vi "Run.vi"(8 "error in (no error)":errorcluster, 11 "AM-AM in":refnum<class "AM-AM.lvclass">) -> (0 "error out":errorcluster, 1 "Parameters":cluster{"Name":string, "Value":string}[](array[cluster]), 2 "Cancled":bool, 3 "AM-AM out":refnum<class "AM-AM.lvclass">)   [LabVIEW 2020, in "AM-AM.lvclass"]
doc: "This is the main test vi. It is here that the test is implemented."
uses:
  AM-AM.lvclass
  C:/Sandbox/RF Bench/Source Code/WiSpry Test Framework/Measurements/Measurement.lvclass
  Controls/Run states.ctl
  Controls/Loop order.ctl
  AM-AM.lvclass/AM-AM.ctl
  Instruments/Spectrum Analyzer/Spectrum Analyzer.lvclass/Spectrum Analyzer.ctl
  Measurement.lvclass/Measurement.ctl
  Devices/Controls/Change setting mode enum.ctl
  Support VI/Update parameters (single).vi
  Devices/Device.lvclass
  Instruments/Spectrum Analyzer/Spectrum Analyzer.lvclass
  Instruments/Signal Generator/Signal Generator.lvclass
  Instruments/Power Meter/Power Meter.lvclass
  Measurement.lvclass
  Devices/PIC-device/PIC-Device.lvclass
  XML Handler/XML Handler.lvclass
panel:
  out "Device Parameters":string
  out "Current Power [dBm]":dbl
  out "Current Frequency [Hz]":dbl format="%#_6p"
  out "Progress":u8(slide) scale=0.0..100.0
  in  "Cancel Button":bool
  out "XY Graph":cluster{dbl[], dbl[]}[](graph)
  out "Estimated finish time":timestamp format="%<%X>T"
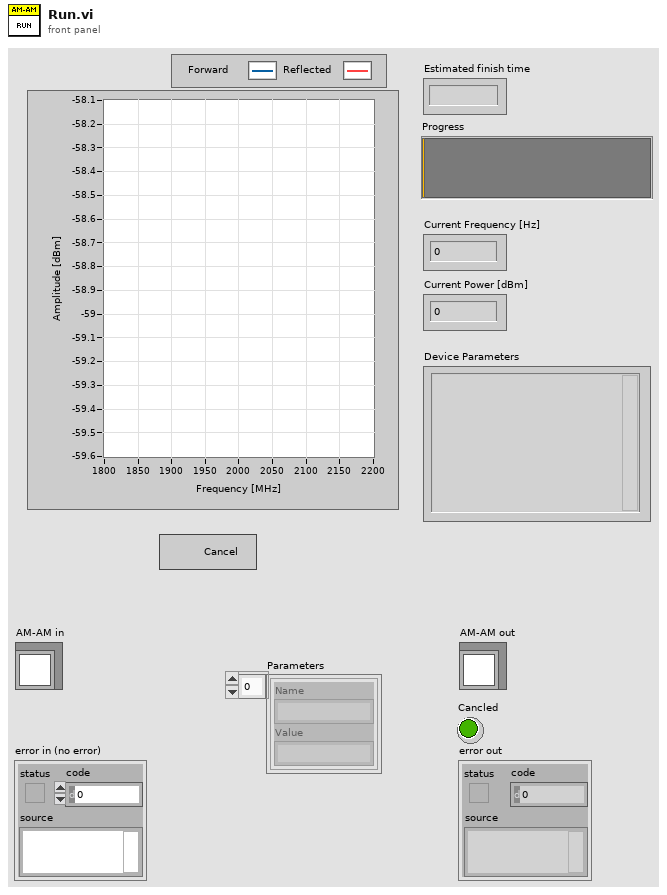
[diagram p1: front panel]
types:
  T1 = typedef "AM-AM.lvclass/Loop order.ctl" = enum16{"Device -> Power -> Frequency", "Device -> Frequency -> Power"}
  T2 = typedef "AM-AM.lvclass/Run states.ctl" = enum16{"Init", "Set Device", "Set Power", "Set Frequency", "Measure", "Done"}
  T3 = typedef "PIC-Device.lvclass/Change setting mode enum.ctl" = enum16{"Init", "Next", "Reset"}
  T4 = typedef "AM-AM.lvclass/Config info.ctl" = cluster{"RBW":dbl, "VBW ":dbl, "Number of Averages":dbl, "Average On":bool, "Power":cluster{"Cluster ":cluster{"From":dbl, "To":dbl, "Step":dbl}, "Array":dbl[], "Use Array":bool}, "Frequency":cluster{"Cluster ":cluster{"From":dbl, "To":dbl, "Step":dbl}, "Array":dbl[], "Use Array":bool}, "Loop order":T1, "Power Window":dbl}
  T5 = typedef "XML Handler.lvclass/Result Cluster.ctl" = cluster{"Name":string, "Value":string}
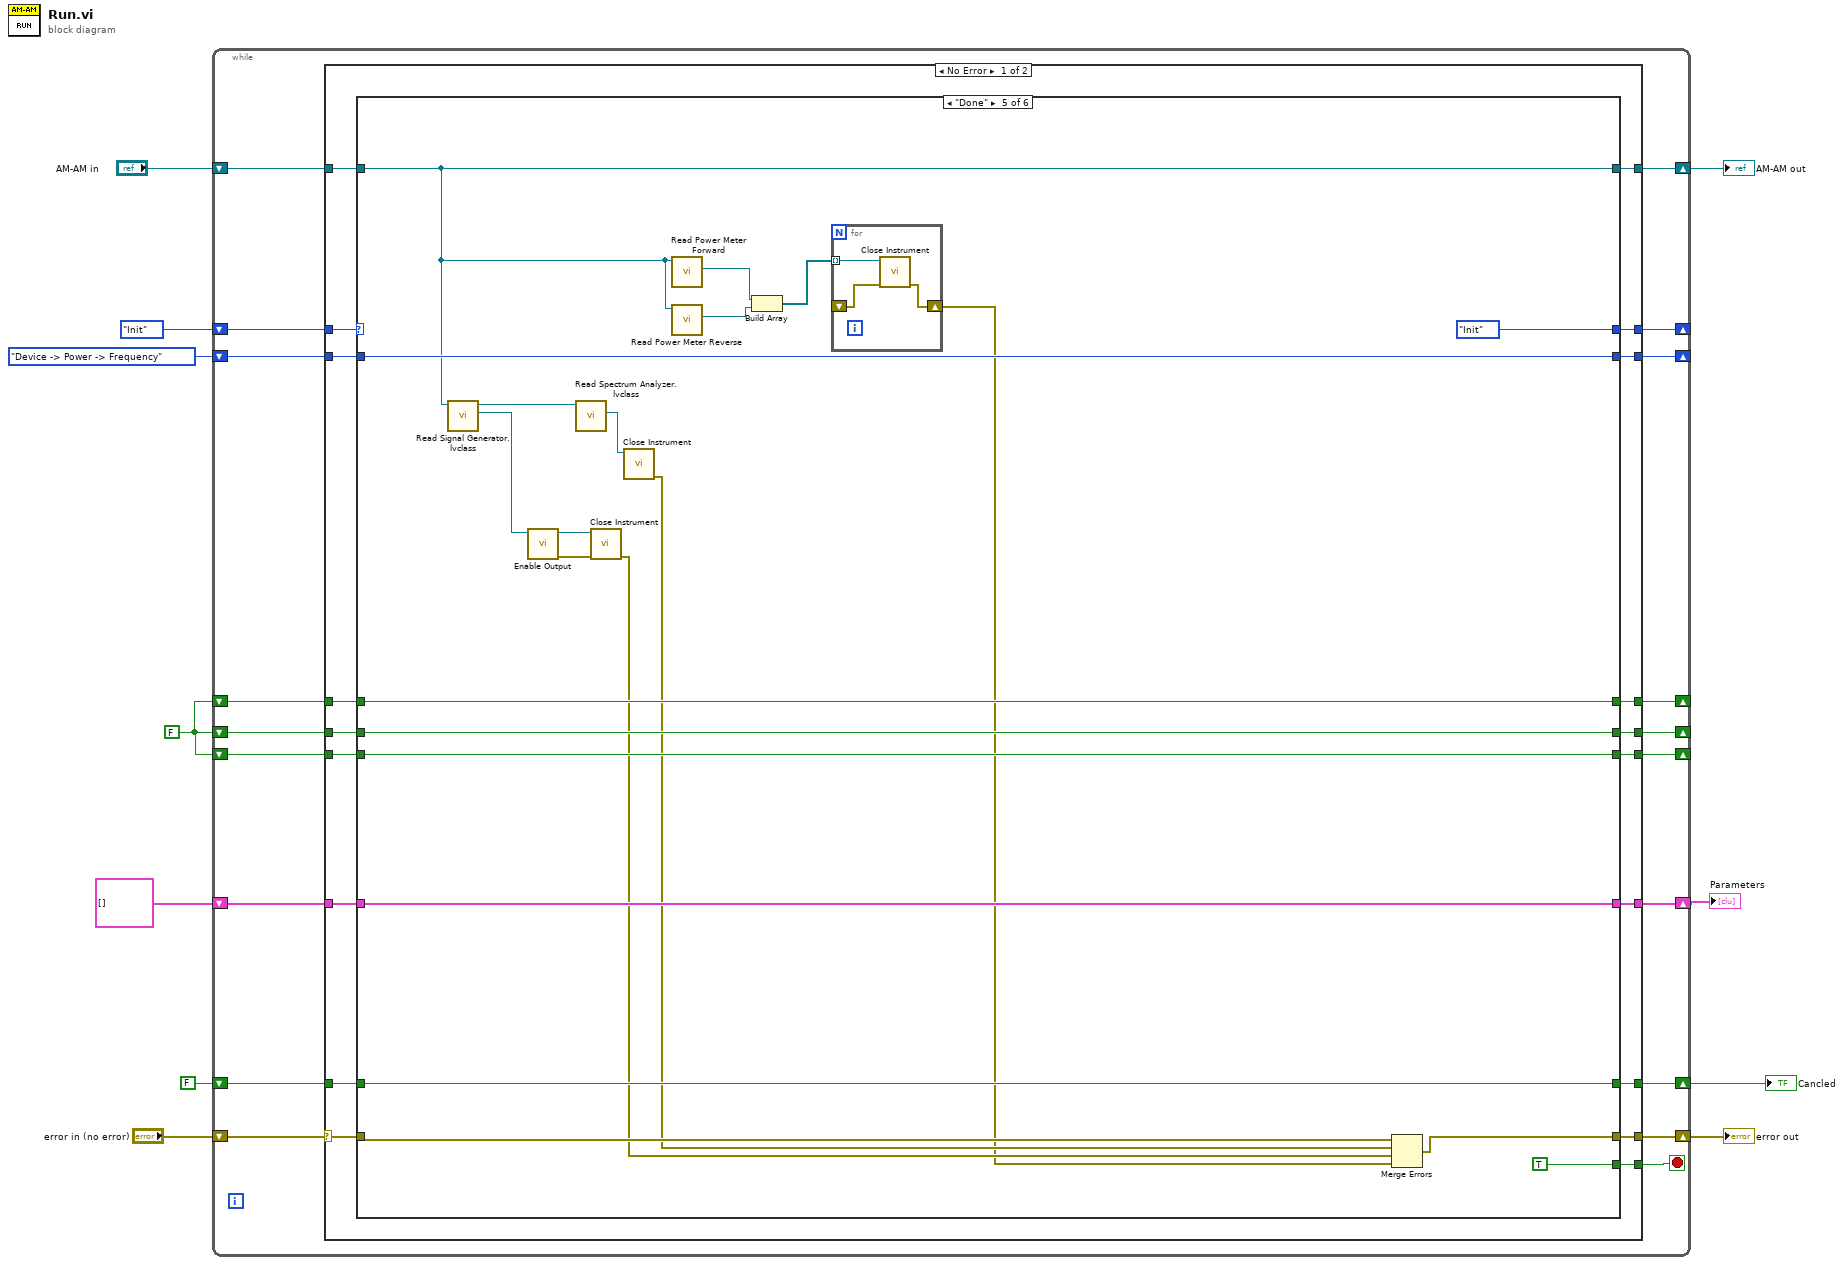
[diagram p0: block diagram]
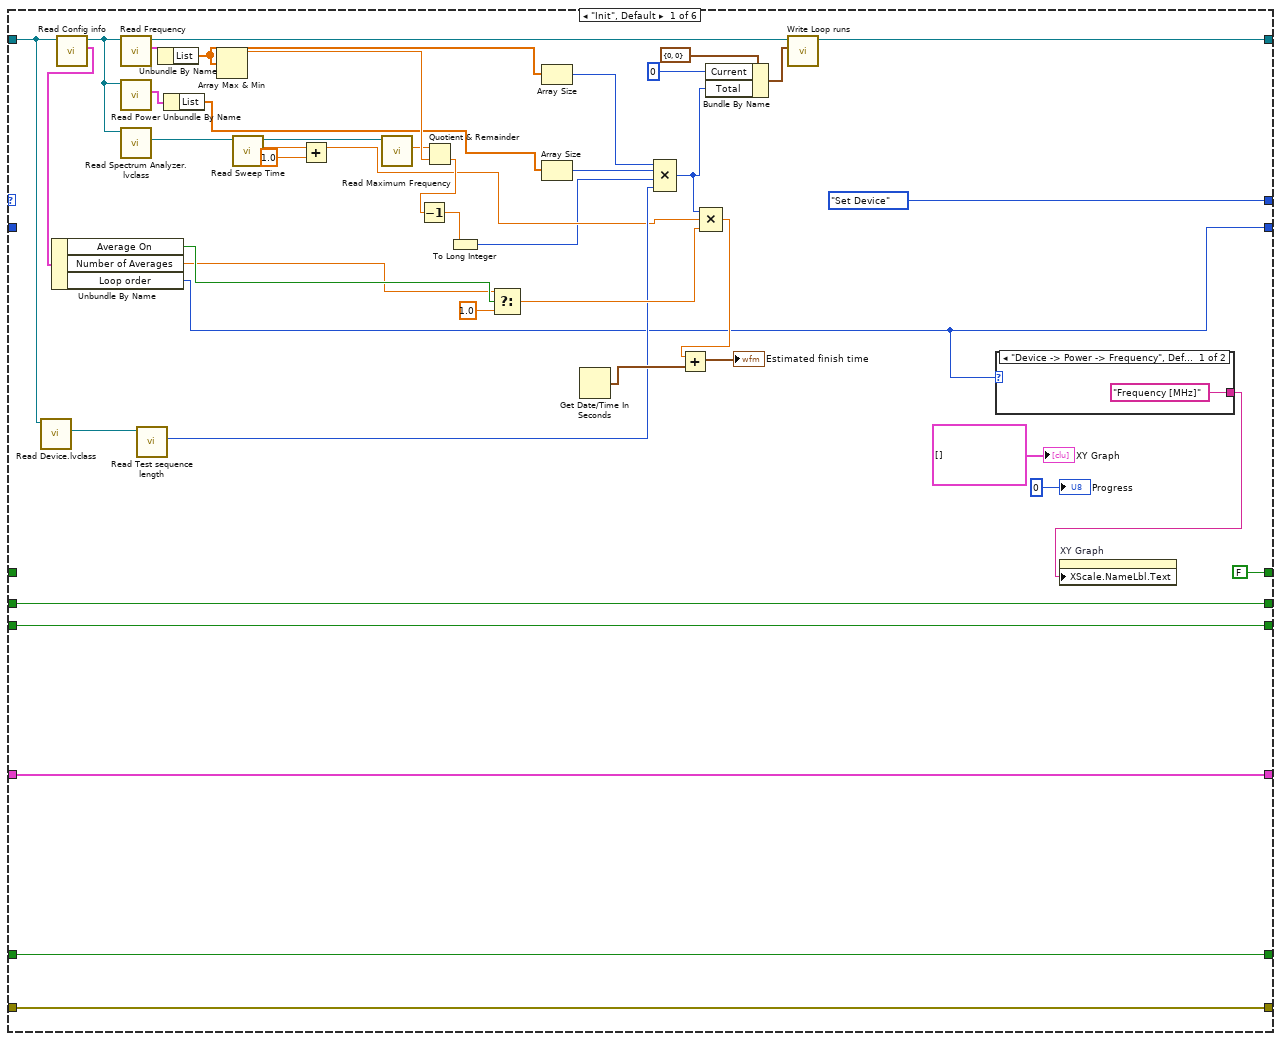
[diagram p2: hidden frame]
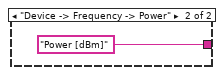
[diagram p3: hidden frame]
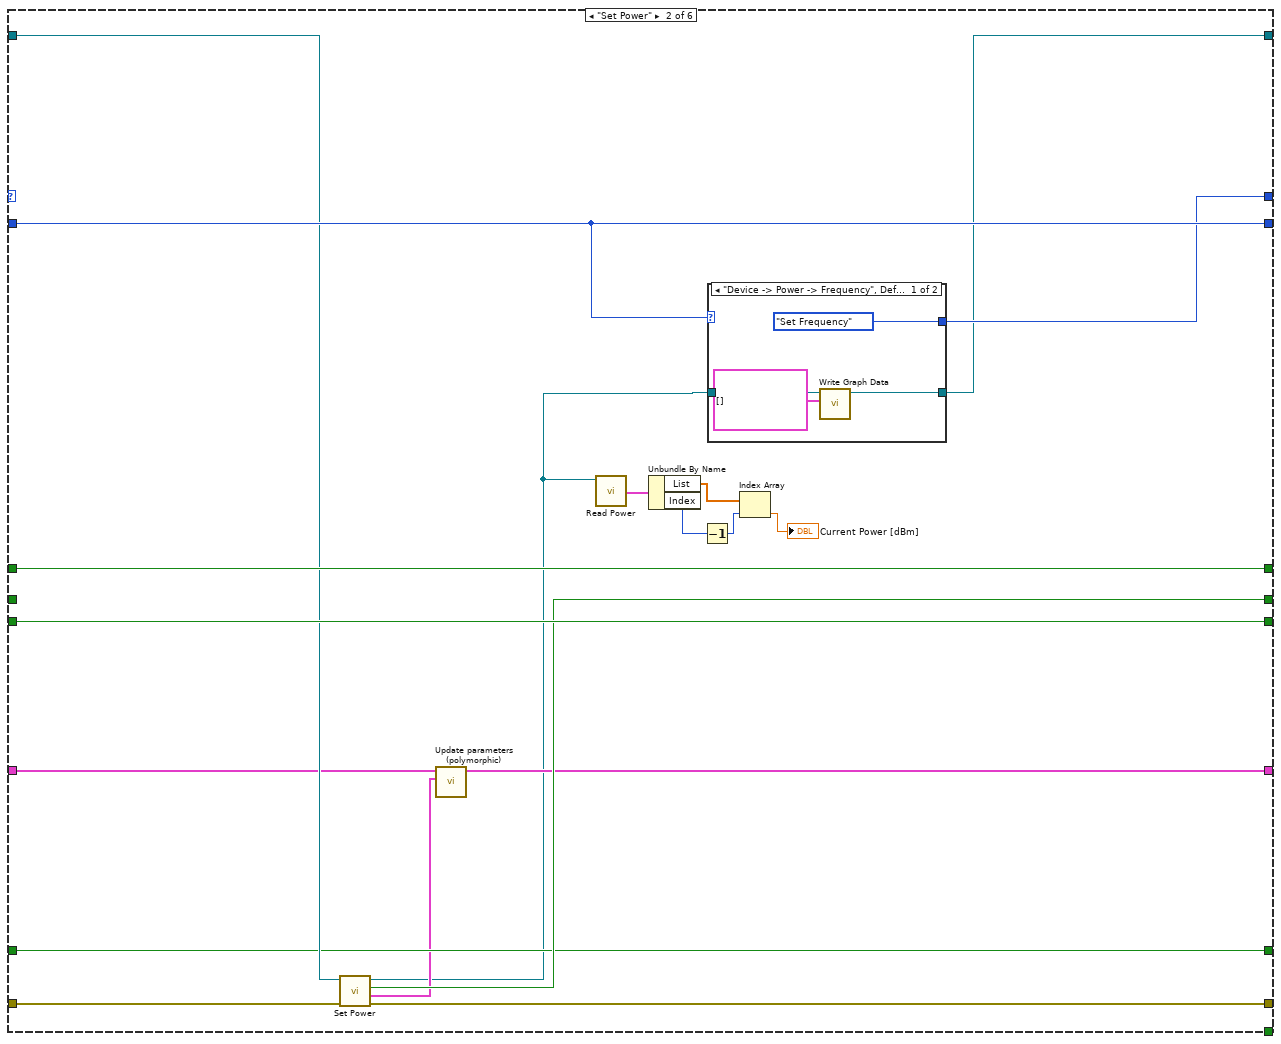
[diagram p4: hidden frame]
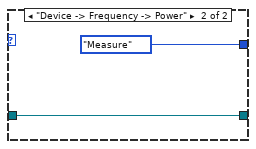
[diagram p5: hidden frame]
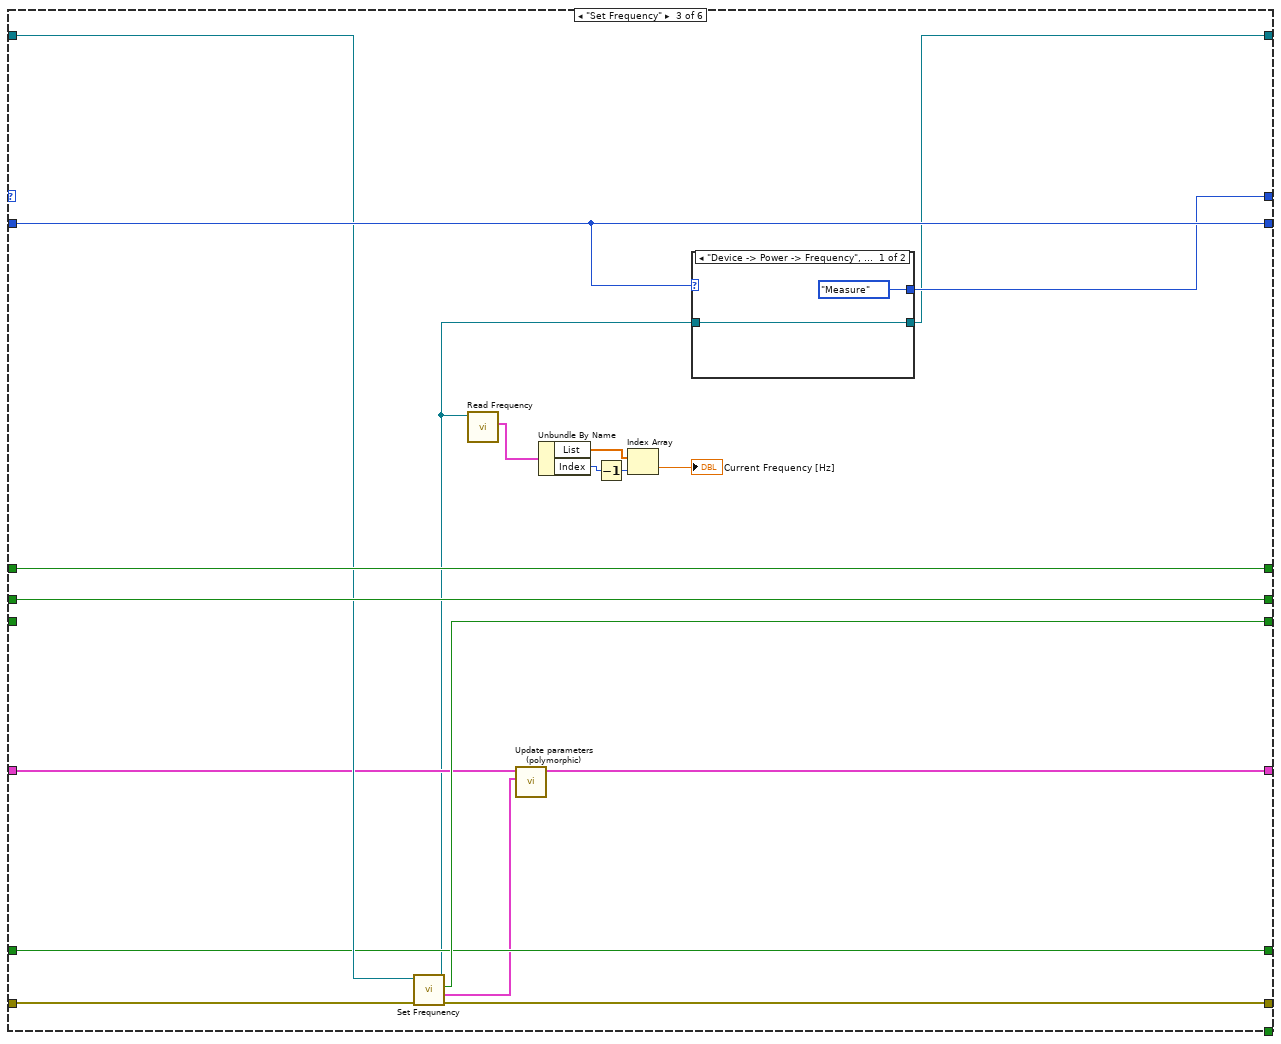
[diagram p6: hidden frame]
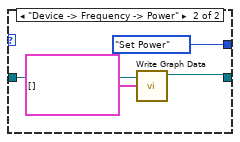
[diagram p7: hidden frame]
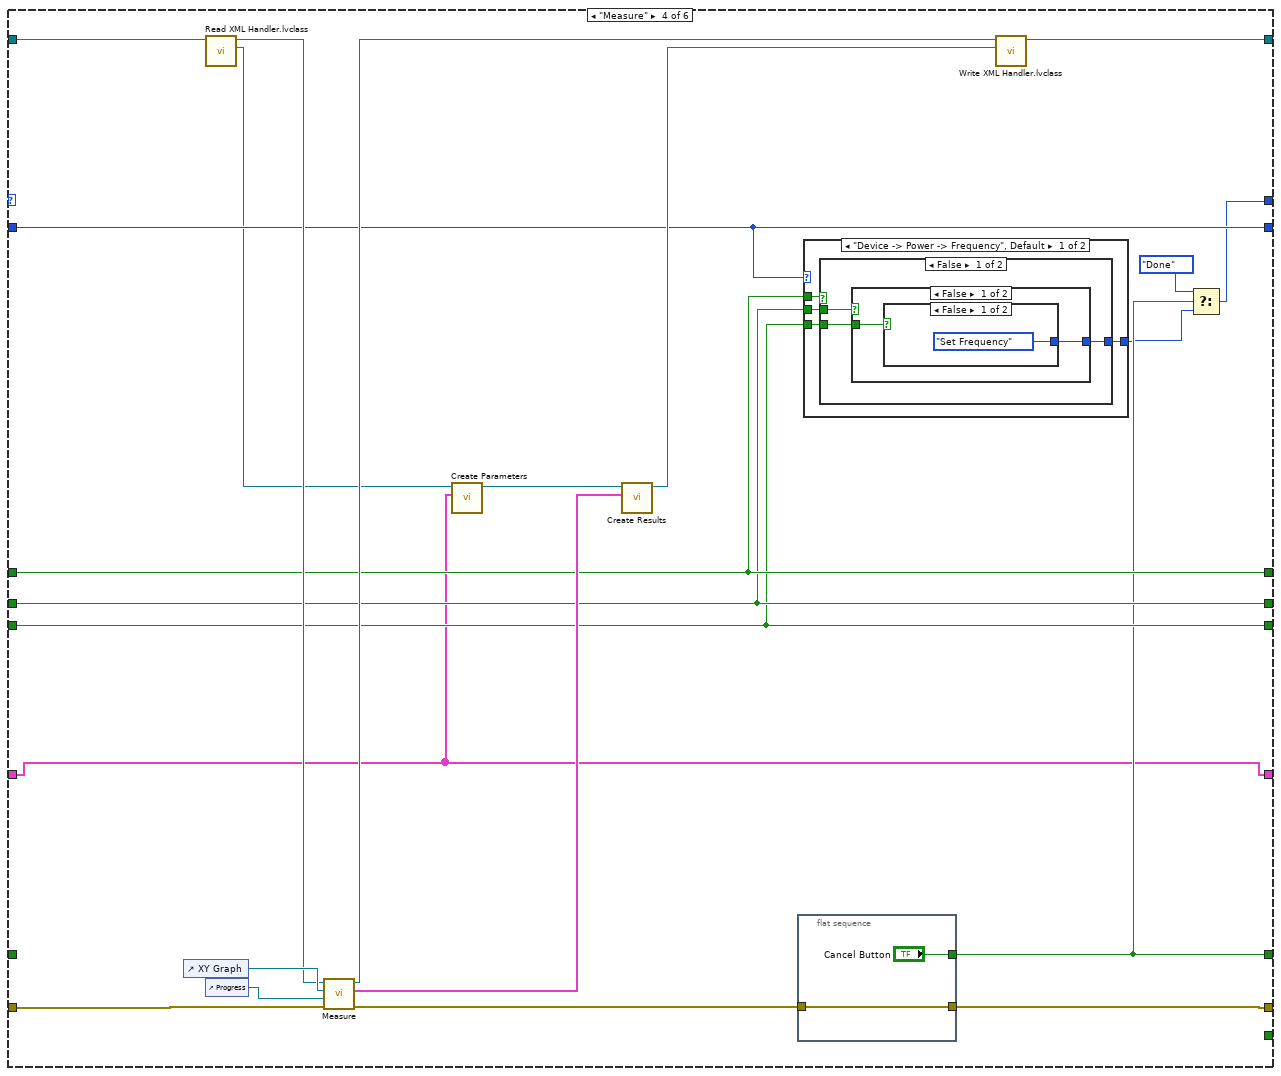
[diagram p8: hidden frame]
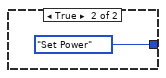
[diagram p9: hidden frame]
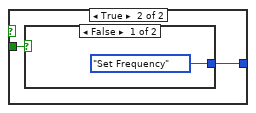
[diagram p10: hidden frame]
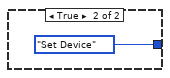
[diagram p11: hidden frame]
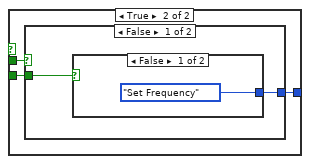
[diagram p12: hidden frame]
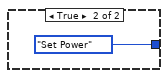
[diagram p13: hidden frame]
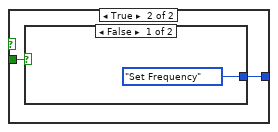
[diagram p14: hidden frame]
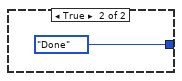
[diagram p15: hidden frame]
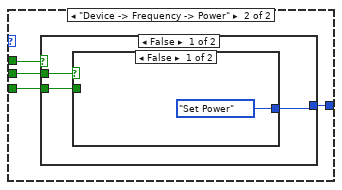
[diagram p16: hidden frame]
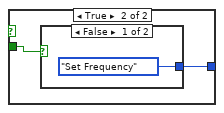
[diagram p17: hidden frame]
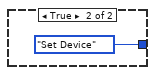
[diagram p18: hidden frame]
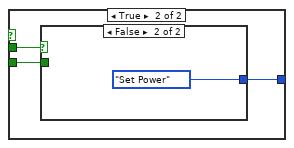
[diagram p19: hidden frame]
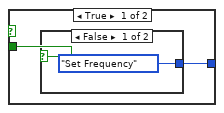
[diagram p20: hidden frame]
diagram:
  w6 = FALSE
  n1 = while {
    shift-right: [w25] -> w8
    shift-left: "error in (no error)" -> [w30]
    shift-right: [w27] -> w9
    shift-left: "AM-AM in" -> [w29]
    shift-right: [w22] -> _
    shift-left: Run_states."Init" ("Run states") -> [w28]
    shift-right: [w24] -> _
    shift-left: w6 -> [w23]
    shift-right: [w21] -> _
    shift-left: Loop_order."Device -> Power -> Frequency" ("Loop order") -> [w20]
    shift-right: [w17] -> _
    shift-left: w6 -> [w19]
    shift-right: [w16] -> _
    shift-left: w6 -> [w18]
    shift-right: [w15] -> w4
    shift-left: FALSE ("Cancel Button") -> [w14]
    shift-right: [w12] -> w1
    shift-left: cluster{"Name":string, "Value":string}[] [] ("Parameters") -> [w13]
    stop <- w26 stop-if-true
    n2 = case shown="No Error" w30 {
      selector: w30 -> [w46 w280]
      tunnel: w29 -> [w49 w281]
      tunnel: w28 -> [w48 _]
      tunnel: [w47 w281] -> w27
      tunnel: [w45 TRUE] -> w26
      tunnel: [w44 w280] -> w25
      tunnel: [w43 _] -> w24
      tunnel: w23 -> [w42 _]
      tunnel: [w41 _] -> w22
      tunnel: [w40 _] -> w21
      tunnel: w20 -> [w39 _]
      tunnel: w19 -> [w38 _]
      tunnel: w18 -> [w37 _]
      tunnel: [w36 _] -> w17
      tunnel: [w35 _] -> w16
      tunnel: [w34 _] -> w15
      tunnel: w14 -> [w33 _]
      tunnel: w13 -> [w32 w279]
      tunnel: [w31 w279] -> w12
      frame No Error {
        n3 = case shown="\"Done\"" w48 {
          tunnel: w49 -> [w79 w110 w135 w166 w220 w266]
          tunnel: [w51 w107 w132 w161 w220 w254] -> w47
          tunnel: w46 -> [w55 w111 w136 w168 w225 w263]
          tunnel: [_ _ _ _ TRUE _] -> w45
          tunnel: [w55 w106 w131 w159 w222 w251] -> w44
          tunnel: [FALSE ("Last setting") w115 w140 w157 w237 w261] -> w43
          tunnel: w42 -> [_ w115 w140 w157 w237 _]
          tunnel: [Run_states."Set Device" ("Run states") w113 w138 w151 Run_states."Init" ("Run states") w257] -> w41
          tunnel: [w57 w114 w139 w158 w238 w258] -> w40
          tunnel: w39 -> [_ w114 w139 w158 w238 w258]
          tunnel: w38 -> [w72 _ w137 w156 w236 w260]
          tunnel: w37 -> [w71 w112 _ w155 w235 w259]
          tunnel: [w72 w109 w137 w156 w236 w260] -> w36
          tunnel: [w71 w112 w134 w155 w235 w259] -> w35
          tunnel: [w66 w108 w133 w154 w232 w256] -> w34
          tunnel: w33 -> [w66 w108 w133 _ w232 w256]
          tunnel: w32 -> [w60 w105 w130 w147 w230 w250]
          tunnel: [w60 w104 w129 w147 w230 w246] -> w31
          frame "Init", Default {
            n4 = call "Read Device.lvclass.vi"("Measurements in"=w79) -> ("Device.lvclass"=w74:refnum<class "Device.lvclass">)  [unwired: 9 in, 1 out]
            n5 = call "Read Config info.vi"("AM-AM in"=w79) -> ("Config info"=w93:T4, "AM-AM out"=w94:refnum<class "AM-AM.lvclass">)  [unwired: 9 in]
            n6 = Unbundle By Name(w93) -> ("Average On"=w84:bool, "Number of Averages"=w83:dbl, "Loop order"=w57:T1)
            n7 = call "Read Frequency.vi"("AM-AM in"=w94) -> ("Frequency"=w70:cluster{"List":dbl[], "Index":i32, "Last":bool}, "AM-AM out"=w65:refnum<class "AM-AM.lvclass">)  [unwired: 9 in]
            n8 = call "Read Power.vi"("AM-AM in"=w94) -> ("Power"=w68:cluster{"List":dbl[], "Index":i32, "Last":bool})  [unwired: 9 in, 1 out]
            n9 = call "Read Spectrum Analyzer.lvclass.vi"("AM-AM in"=w94) -> ("Spectrum Analyzer.lvclass"=w92:refnum<class "Spectrum Analyzer.lvclass">)  [unwired: 9 in, 1 out]
            n10 = call-dynamic "Read Test sequence length.vi"("Device in"=w74) -> ("Test sequence length"=w75:i32)  [unwired: 8 in, 2 out]
            n11 = Unbundle By Name(w70) -> ("List"=w69:dbl[])
            n12 = Unbundle By Name(w68) -> ("List"=w67:dbl[])
            n13 = Array Max & Min(array=w69) -> (max value=w90:dbl)  [unwired: 3 out]
            n14 = call "Read Sweep Time.vi"("Spectrum Analyzer in"=w92) -> ("Sweep Time"=w87:dbl, "Spectrum Analyzer out"=w91:refnum<class "Spectrum Analyzer.lvclass">)  [unwired: 9 in]
            n15 = Add(x=w87, y=1.0) -> (x+y=w53:dbl)
            n16 = call "Read Maximum Frequency.vi"("Spectrum Analyzer in"=w91) -> ("Maximum Frequency"=w89:dbl)  [unwired: 9 in, 1 out]
            n17 = Quotient & Remainder(x=w89, y=w90) -> (floor(x/y)=w88:dbl)  [unwired: 1 out]
            n18 = Decrement(x=w88) -> (x-1=w80:dbl)
            n19 = To Long Integer(number=w80) -> (32bit integer=w50:i32)
            n20 = Select(t=w83, s=w84, f=1.0) -> (s? t:f=w81:dbl)
            n21 = Array Size(array=w69) -> (size(s)=w77:i32)
            n22 = Array Size(array=w67) -> (size(s)=w76:i32)
            n23 = Get Date/Time In Seconds() -> (seconds since 1Jan1904=w86:timestamp)
            n24 = Compound Arithmetic op=MULTIPLY(w77, w76, w50, w75) -> (w61:i32)
            n25 = Compound Arithmetic op=MULTIPLY(w61, w53, w81) -> (w78:dbl)
            n26 = Add(x=w78, y=w86) -> (x+y=→"Estimated finish time":timestamp)
            n27 = Bundle By Name(cluster=cluster{"Current":u32, "Total":u32} {"Current"=0, "Total"=0} ("Loop runs"), "Current"=u32 0, "Total"=w61) -> (w62:cluster{"Current":u32, "Total":u32})
            n28 = call "Write Loop runs.vi"("Loop runs"=w62, "Measurements in"=w65) -> ("Measurements out"=w51:refnum<class "AM-AM.lvclass">)  [unwired: 9 in]
            n29 = case shown="\"Device -> Power -> Frequency\", Default" w57 {
              tunnel: ["Frequency [MHz]" "Power [dBm]"] -> w56
              frame "Device -> Power -> Frequency", Default {
              }
              frame "Device -> Frequency -> Power" {
              }
            }
            n30 = property on="XY Graph" class="XYGraph (strict)"("XScale.NameLbl.Text"=w56) -> ()  [unwired: 2 in, 2 out]
            "XY Graph" <- cluster{dbl[], dbl[]}[] [] ("XY Graph")
            "Progress" <- u8 0 ("Progress")
          }
          frame "Set Power" {
            n31 = call "Set Power.vi"("error in (no error)"=w111, "AM-AM in"=w110) -> ("error out"=w106:errorcluster, "Parameter"=w103:cluster{"Name":string, "Value":string}, "Last Power?"=w109:bool, "AM-AM out"=w102:refnum<class "AM-AM.lvclass">)  [unwired: 6 in]
            n32 = call-poly "Update parameters (polymorphic).vi"("New Parameter"=w103, "Parameters"=w105) -> ("Parameters Out"=w104:cluster{"Name":string, "Value":string}[])  [unwired: 9 in]
            n33 = call "Read Power.vi"("AM-AM in"=w102) -> ("Power"=w101:cluster{"List":dbl[], "Index":i32, "Last":bool})  [unwired: 9 in, 1 out]
            n34 = Unbundle By Name(w101) -> ("List"=w99:dbl[], "Index"=w97:i32)
            n35 = Decrement(x=w97) -> (x-1=w98:i32)
            n36 = case shown="\"Device -> Power -> Frequency\", Default" w114 {
              tunnel: [Run_states."Set Frequency" ("Run states") Run_states."Measure" ("Run states")] -> w113
              tunnel: w102 -> [w118 w120]
              tunnel: [w117 w120] -> w107
              frame "Device -> Power -> Frequency", Default {
                n37 = call "Write Graph Data.vi"("Graph Data"=cluster{"Array":dbl[], "Array":dbl[]}[] [], "AM-AM in"=w118) -> ("AM-AM out"=w117:refnum<class "AM-AM.lvclass">)  [unwired: 9 in]
              }
              frame "Device -> Frequency -> Power" {
              }
            }
            n38 = Index Array(array=w99, index=w98) -> (element=→"Current Power [dBm]":dbl)
          }
          frame "Set Frequency" {
            n39 = call "Set Frequnency.vi"("error in (no error)"=w136, "AM-AM in"=w135) -> ("error out"=w131:errorcluster, "Parameter"=w128:cluster{"Name":string, "Value":string}, "Last Frequency?"=w134:bool, "AM-AM out"=w127:refnum<class "AM-AM.lvclass">)  [unwired: 6 in]
            n40 = call "Read Frequency.vi"("AM-AM in"=w127) -> ("Frequency"=w126:cluster{"List":dbl[], "Index":i32, "Last":bool})  [unwired: 9 in, 1 out]
            n41 = call-poly "Update parameters (polymorphic).vi"("New Parameter"=w128, "Parameters"=w130) -> ("Parameters Out"=w129:cluster{"Name":string, "Value":string}[])  [unwired: 9 in]
            n42 = Unbundle By Name(w126) -> ("List"=w125:dbl[], "Index"=w124:i32)
            n43 = Decrement(x=w124) -> (x-1=w123:i32)
            n44 = Index Array(array=w125, index=w123) -> (element=→"Current Frequency [Hz]":dbl)
            n45 = case shown="\"Device -> Power -> Frequency\", Default" w139 {
              tunnel: [Run_states."Measure" ("Run states") Run_states."Set Power" ("Run states")] -> w138
              tunnel: [w141 w144] -> w132
              tunnel: w127 -> [w141 w145]
              frame "Device -> Power -> Frequency", Default {
              }
              frame "Device -> Frequency -> Power" {
                n46 = call "Write Graph Data.vi"("Graph Data"=cluster{"Array":dbl[], "Array":dbl[]}[] [], "AM-AM in"=w145) -> ("AM-AM out"=w144:refnum<class "AM-AM.lvclass">)  [unwired: 9 in]
              }
            }
          }
          frame "Measure" {
            n47 = control-ref of="XY Graph"() -> (w164:refnum<vi>)
            n48 = call "Read XML Handler.lvclass.vi"("Measurements in"=w166) -> ("XML Handler.lvclass"=w149:refnum<class "XML Handler.lvclass">, "Measurements out"=w163:refnum<class "AM-AM.lvclass">)  [unwired: 9 in]
            n49 = control-ref of="Progress"() -> (w150:refnum<vi>)
            n50 = call "Measure.vi"("error in (no error)"=w168, "Progress Ref"=w150, "XY Graph Reference"=w164, "AM-AM in"=w163) -> ("error out"=w160:errorcluster, "Results"=w167:T5[], "AM-AM out"=w162:refnum<class "AM-AM.lvclass">)  [unwired: 5 in]
            n51 = call "Create Parameters.vi"("Parameters"=w147, "XML Handler in"=w149) -> ("XML Handler out"=w148:refnum<class "XML Handler.lvclass">)  [unwired: 8 in, 1 out]
            n52 = call "Create Results.vi"("Results"=w167, "XML Handler in"=w148) -> ("XML Handler out"=w165:refnum<class "XML Handler.lvclass">)  [unwired: 8 in, 1 out]
            n53 = flat-sequence {
              tunnel: w160 -> [w216]
              tunnel: [w216] -> w159
              tunnel: ["Cancel Button"] -> w154
              frame #0 {
              }
            }
            n54 = case shown="\"Device -> Power -> Frequency\", Default" w158 {
              tunnel: w157 -> [w172 w198]
              tunnel: w156 -> [w171 w197]
              tunnel: w155 -> [w170 w196]
              tunnel: [w169 w195] -> w153
              frame "Device -> Power -> Frequency", Default {
                n55 = case shown="False" w172 {
                  tunnel: w171 -> [w175 w186]
                  tunnel: w170 -> [w174 w185]
                  tunnel: [w173 w184] -> w169
                  frame False {
                    n56 = case shown="False" w175 {
                      tunnel: w174 -> [w177 w181]
                      tunnel: [w176 w180] -> w173
                      frame False {
                        n57 = case shown="False" w177 {
                          tunnel: [Run_states."Set Frequency" ("Run states") Run_states."Set Power" ("Run states")] -> w176
                          frame False {
                          }
                          frame True {
                          }
                        }
                      }
                      frame True {
                        n58 = case shown="False" w181 {
                          tunnel: [Run_states."Set Frequency" ("Run states") Run_states."Set Device" ("Run states")] -> w180
                          frame False {
                          }
                          frame True {
                          }
                        }
                      }
                    }
                  }
                  frame True {
                    n59 = case shown="False" w186 {
                      tunnel: w185 -> [w188 w192]
                      tunnel: [w187 w191] -> w184
                      frame False {
                        n60 = case shown="False" w188 {
                          tunnel: [Run_states."Set Frequency" ("Run states") Run_states."Set Power" ("Run states")] -> w187
                          frame False {
                          }
                          frame True {
                          }
                        }
                      }
                      frame True {
                        n61 = case shown="False" w192 {
                          tunnel: [Run_states."Set Frequency" ("Run states") Run_states."Done" ("Run states")] -> w191
                          frame False {
                          }
                          frame True {
                          }
                        }
                      }
                    }
                  }
                }
              }
              frame "Device -> Frequency -> Power" {
                n62 = case shown="False" w198 {
                  tunnel: w197 -> [w201 w209]
                  tunnel: w196 -> [w200 w208]
                  tunnel: [w199 w207] -> w195
                  frame False {
                    n63 = case shown="False" w201 {
                      tunnel: w200 -> [_ w204]
                      tunnel: [Run_states."Set Power" ("Run states") w203] -> w199
                      frame False {
                      }
                      frame True {
                        n64 = case shown="False" w204 {
                          tunnel: [Run_states."Set Frequency" ("Run states") Run_states."Set Device" ("Run states")] -> w203
                          frame False {
                          }
                          frame True {
                          }
                        }
                      }
                    }
                  }
                  frame True {
                    n65 = case shown="False" w209 {
                      tunnel: w208 -> [w211 _]
                      tunnel: [w210 Run_states."Set Power" ("Run states")] -> w207
                      frame True {
                        n66 = case shown="False" w211 {
                          tunnel: [Run_states."Set Frequency" ("Run states") Run_states."Done" ("Run states")] -> w210
                          frame False {
                          }
                          frame True {
                          }
                        }
                      }
                      frame False {
                      }
                    }
                  }
                }
              }
            }
            n67 = call "Write XML Handler.lvclass.vi"("XML Handler.lvclass"=w165, "Measurements in"=w162) -> ("Measurements out"=w161:refnum<class "AM-AM.lvclass">)  [unwired: 9 in]
            n68 = Select(t=Run_states."Done", s=w154, f=w153) -> (s? t:f=w151:T2)
          }
          frame "Done" {
            n69 = call "Read Signal Generator.lvclass.vi"("AM-AM in"=w220) -> ("Signal Generator.lvclass"=w231:refnum<class "Signal Generator.lvclass">, "AM-AM out"=w229:refnum<class "AM-AM.lvclass">)  [unwired: 9 in]
            n70 = call-dynamic "Enable Output.vi"("Signal Generator in"=w231) -> ("error out"=w227:errorcluster, "Signal Generator out"=w228:refnum<class "Signal Generator.lvclass">)  [unwired: 9 in]
            n71 = call "Read Spectrum Analyzer.lvclass.vi"("AM-AM in"=w229) -> ("Spectrum Analyzer.lvclass"=w226:refnum<class "Spectrum Analyzer.lvclass">)  [unwired: 9 in, 1 out]
            n72 = call-dynamic "Close Instrument.vi"("error in (no error)"=w227, "Instrument in"=w228) -> ("error out"=w223:errorcluster)  [unwired: 8 in, 1 out]
            n73 = call-dynamic "Close Instrument.vi"("Instrument in"=w226) -> ("error out"=w224:errorcluster)  [unwired: 9 in, 1 out]
            n74 = call "Read Power Meter Forward.vi"("AM-AM in"=w220) -> ("Power Meter Forward"=w219:refnum<class "Power Meter.lvclass">)  [unwired: 9 in, 1 out]
            n75 = call "Read Power Meter Reverse.vi"("AM-AM in"=w220) -> ("Power Meter.lvclass"=w218:refnum<class "Power Meter.lvclass">)  [unwired: 9 in, 1 out]
            n76 = Build Array(w219, w218) -> (w217:refnum<class "Power Meter.lvclass">[])
            n77 = for {
              shift-right: [w241] -> w221
              shift-left: _ -> [w240]
              tunnel: w217 -> [w239] mode=indexing
              n78 = call-dynamic "Close Instrument.vi"("error in (no error)"=w240, "Instrument in"=w239) -> ("error out"=w241:errorcluster)  [unwired: 8 in, 1 out]
            }
            n79 = Merge Errors(w225, w224, w223, w221) -> (w222:errorcluster)
          }
          frame "Set Device" {
            n80 = call "Read Device.lvclass.vi"("Measurements in"=w266) -> ("Device.lvclass"=w265:refnum<class "Device.lvclass">, "Measurements out"=w255:refnum<class "AM-AM.lvclass">)  [unwired: 9 in]
            n81 = call-dynamic "Change Setting.vi"("error in (no error)"=w263, "Change setting mode"=Change_setting_mode_enum."Next", "Device in"=w265) -> ("error out"=w251:errorcluster, "Changes"=w249:cluster{"Name":string, "Value":string}[], "Last setting"=w261:bool, "Device out"=w262:refnum<class "Device.lvclass">)  [unwired: 5 in]
            n82 = call "Write Device.lvclass.vi"("Device.lvclass"=w262, "Measurements in"=w255) -> ("Measurements out"=w252:refnum<class "AM-AM.lvclass">)  [unwired: 9 in]
            n83 = for {
              shift-right: [w275] -> w246
              shift-left: w250 -> [w276]
              tunnel: w249 -> [w274] mode=indexing
              n84 = call-poly "Update parameters (polymorphic).vi"("New Parameter"=w274, "Parameters"=w276) -> ("Parameters Out"=w275:cluster{"Name":string, "Value":string}[])  [unwired: 9 in]
            }
            n85 = Array Size(array=w249) -> (size(s)=w247:i32)
            n86 = Decrement(x=w247) -> (x-1=w242:i32)
            n87 = Array Subset(array=w246, index=0, length=w242) -> (w245:cluster{"Name":string, "Value":string}[])
            n88 = call "Write Graph Data.vi"("Graph Data"=cluster{"Array":dbl[], "Array":dbl[]}[] [], "AM-AM in"=w252) -> ("AM-AM out"=w254:refnum<class "AM-AM.lvclass">)  [unwired: 9 in]
            n89 = for {
              tunnel: w245 -> [w273] mode=indexing
              shift-right: [w267] -> w243
              shift-left: "" -> [w272]
              n90 = Unbundle By Name(w273) -> ("Name"=w271:string, "Value"=w269:string)
              n91 = Concatenate Strings(w272, w271, ": " ("string"), w269, "\r\n") -> (w267:string)
            }
            "Device Parameters" <- w243
            n92 = case shown="\"Device -> Power -> Frequency\", Default" w258 {
              tunnel: [Run_states."Set Power" ("Run states") Run_states."Set Frequency" ("Run states")] -> w257
              frame "Device -> Power -> Frequency", Default {
              }
              frame "Device -> Frequency -> Power" {
              }
            }
          }
        }
      }
      frame Error {
      }
    }
  }
  "error out" <- w8
  "AM-AM out" <- w9
  "Cancled" <- w4
  "Parameters" <- w1
